vi "Populate.vi"(8 "error in":errorcluster, 9 "Values In":string[](array[string]), 10 "Keys In":string[](array[string]), 11 "Fast Tree in":refnum<class "Fast Tree.lvclass">) -> (0 "error out":errorcluster, 2 "Tree Out":T1(array[cluster]), 3 "Fast Tree out":refnum<class "Fast Tree.lvclass">)   [LabVIEW 2019, in "Fast Tree.lvclass"]
uses:
  Fast Tree.lvclass
  Fast Tree.lvclass/Fast Tree.ctl
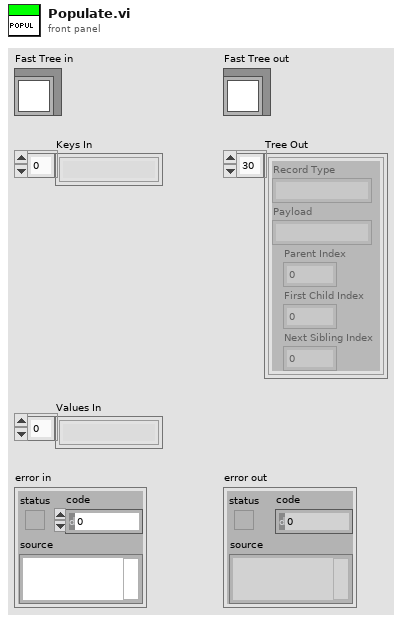
[diagram p1: front panel]
types:
  T1 = cluster{"Record Type":string, "Payload":string, "Parent Index":i32, "First Child Index":i32, "Next Sibling Index":i32}[]
  T2 = cluster{"Record Type":string, "Payload":string, "Parent Index":i32, "First Child Index":i32, "Next Sibling Index":i32}
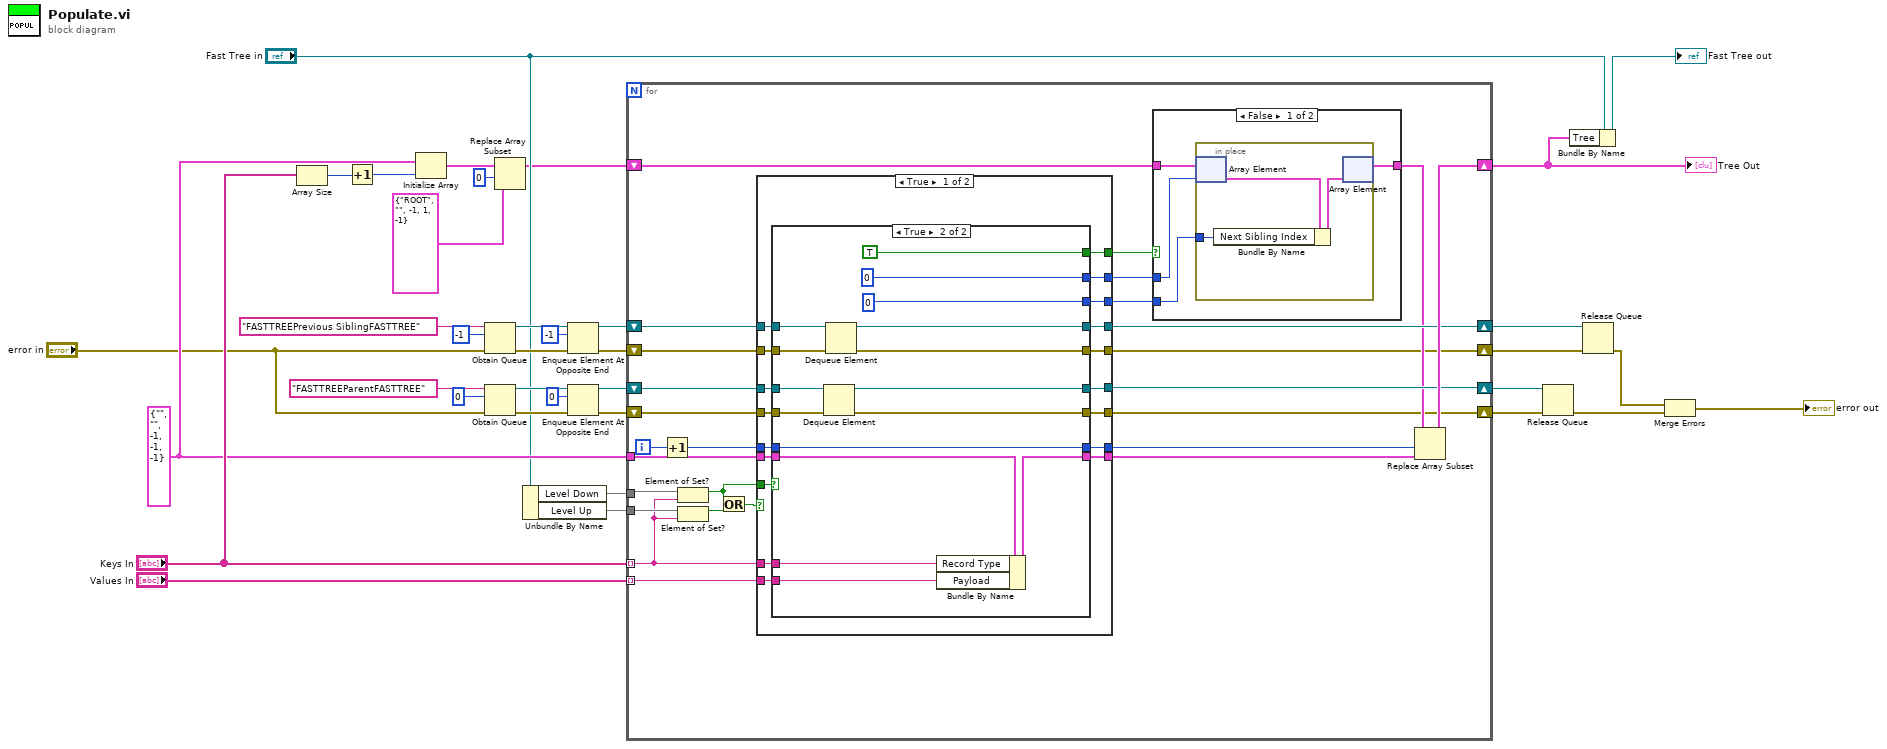
[diagram p0: block diagram]
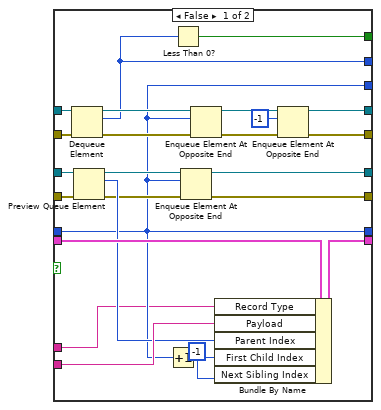
[diagram p3: hidden frame]
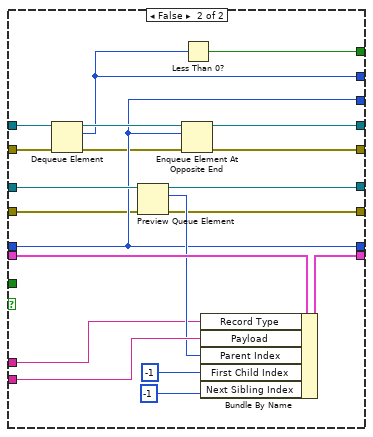
[diagram p4: hidden frame]
diagram:
  w17 = T2 {"Record Type"="", "Payload"="", "Parent Index"=-1, "First Child Index"=-1, "Next Sibling Index"=-1} ("Node")
  n1 = Array Size(array="Keys In") -> (size(s)=w18:i32)
  n2 = Increment(x=w18) -> (x+1=w11:i32)
  n3 = Initialize Array(w17, w11) -> (w10:T1)
  n4 = Obtain Queue(name (unnamed)="FASTTREEPrevious SiblingFASTTREE", element data type=-1, error in (no error)="error in") -> (queue out=w30:refnum<queue>, error out=w23:errorcluster)  [unwired: 2 in, 1 out]
  n5 = Obtain Queue(name (unnamed)="FASTTREEParentFASTTREE", element data type=0, error in (no error)="error in") -> (queue out=w32:refnum<queue>, error out=w22:errorcluster)  [unwired: 2 in, 1 out]
  n6 = Replace Array Subset(array=w10, new element=T2 {"Record Type"="ROOT", "Payload"="", "Parent Index"=-1, "First Child Index"=1, "Next Sibling Index"=-1} ("Node"), index=0) -> (w9:T1)
  n7 = Unbundle By Name("Fast Tree in") -> ("Level Down"=w15:set{string}, "Level Up"=w16:set{string})
  n8 = Enqueue Element At Opposite End(queue=w30, element=-1, error in (no error)=w23) -> (queue out=w26:refnum<queue>, error out=w24:errorcluster)  [unwired: 1 in, 1 out]
  n9 = Enqueue Element At Opposite End(queue=w32, element=0, error in (no error)=w22) -> (queue out=w31:refnum<queue>, error out=w21:errorcluster)  [unwired: 1 in, 1 out]
  n10 = for {
    shift-right: [w57] -> w12
    shift-left: w9 -> [w38]
    tunnel: "Keys In" -> [w40] mode=indexing
    tunnel: "Values In" -> [w61] mode=indexing
    tunnel: w17 -> [w62]
    shift-right: [w54] -> w35
    shift-left: w31 -> [w55]
    shift-right: [w52] -> w25
    shift-left: w26 -> [w53]
    shift-right: [w47] -> w5
    shift-left: w21 -> [w46]
    shift-right: [w45] -> w4
    shift-left: w24 -> [w44]
    tunnel: w16 -> [w43]
    tunnel: w15 -> [w42]
    i -> [w59]
    n11 = Increment(x=w59) -> (x+1=w58:i32)
    n12 = Element of Set?(10:w40, 11:w42) -> (3:w37:bool)
    n13 = Element of Set?(10:w40, 11:w43) -> (3:w41:bool)
    n14 = Or(x=w37, y=w41) -> (x .or. y?=w39:bool)
    n15 = case shown="True" w39 {
      tunnel: w62 -> [w86 w147]
      tunnel: w61 -> [w85 w146]
      tunnel: w58 -> [w79 w137]
      tunnel: [w87 w148] -> w60
      tunnel: [w73 w137] -> w56
      tunnel: w55 -> [w84 w145]
      tunnel: [w88 w140] -> w54
      tunnel: w53 -> [w83 w141]
      tunnel: [w82 w139] -> w52
      tunnel: [w81 w138] -> w48
      tunnel: [w80 w135] -> w50
      tunnel: [w72 w137] -> w49
      tunnel: [w77 w131] -> w47
      tunnel: w46 -> [w78 w130]
      tunnel: [w76 w132] -> w45
      tunnel: w44 -> [w75 w134]
      tunnel: w40 -> [w71 w129]
      tunnel: w37 -> [w74 _]
      frame True {
        n16 = case shown="True" w74 {
          tunnel: [w112 w118] -> w88
          tunnel: [w111 w116] -> w87
          tunnel: w86 -> [w110 w115]
          tunnel: w85 -> [w109 w113]
          tunnel: w84 -> [w107 w119]
          tunnel: w83 -> [w103 w128]
          tunnel: [w101 w125] -> w82
          tunnel: [w99 TRUE] -> w81
          tunnel: [w98 0] -> w80
          tunnel: w79 -> [w90 w122]
          tunnel: w78 -> [w96 w120]
          tunnel: [w94 w121] -> w77
          tunnel: [w93 w126] -> w76
          tunnel: w75 -> [w91 w127]
          tunnel: [w90 w122] -> w73
          tunnel: [w90 0] -> w72
          tunnel: w71 -> [w89 w114]
          frame False {
            n17 = Dequeue Element(queue=w103, error in (no error)=w91) -> (queue out=w104:refnum<queue>, element=w98:i32, error out=w92:errorcluster)  [unwired: 1 in, 1 out]
            n18 = Preview Queue Element(queue=w107, error in (no error)=w96) -> (queue out=w108:refnum<queue>, element=w97:i32, error out=w95:errorcluster)  [unwired: 1 in, 1 out]
            n19 = Increment(x=w90) -> (x+1=w106:i32)
            n20 = Less Than 0?(x=w98) -> (x < 0?=w99:bool)
            n21 = Enqueue Element At Opposite End(queue=w108, element=w90, error in (no error)=w95) -> (queue out=w112:refnum<queue>, error out=w94:errorcluster)  [unwired: 1 in, 1 out]
            n22 = Enqueue Element At Opposite End(queue=w104, element=w90, error in (no error)=w92) -> (queue out=w102:refnum<queue>, error out=w93:errorcluster)  [unwired: 1 in, 1 out]
            n23 = Bundle By Name(cluster=w110, "Record Type"=w89, "Payload"=w109, "Parent Index"=w97, "First Child Index"=w106, "Next Sibling Index"=-1) -> (w111:T2)
            n24 = Enqueue Element At Opposite End(queue=w102, element=-1) -> (queue out=w101:refnum<queue>)  [unwired: 2 in, 2 out]
          }
          frame True {
            n25 = Dequeue Element(queue=w119, error in (no error)=w120) -> (queue out=w118:refnum<queue>, error out=w121:errorcluster)  [unwired: 1 in, 2 out]
            n26 = Dequeue Element(queue=w128, error in (no error)=w127) -> (queue out=w125:refnum<queue>, error out=w126:errorcluster)  [unwired: 1 in, 2 out]
            n27 = Bundle By Name(cluster=w115, "Record Type"=w114, "Payload"=w113) -> (w116:T2)
          }
        }
      }
      frame False {
        n28 = Dequeue Element(queue=w141, error in (no error)=w134) -> (queue out=w142:refnum<queue>, element=w135:i32, error out=w133:errorcluster)  [unwired: 1 in, 1 out]
        n29 = Preview Queue Element(queue=w145, error in (no error)=w130) -> (queue out=w140:refnum<queue>, element=w144:i32, error out=w131:errorcluster)  [unwired: 1 in, 1 out]
        n30 = Enqueue Element At Opposite End(queue=w142, element=w137, error in (no error)=w133) -> (queue out=w139:refnum<queue>, error out=w132:errorcluster)  [unwired: 1 in, 1 out]
        n31 = Less Than 0?(x=w135) -> (x < 0?=w138:bool)
        n32 = Bundle By Name(cluster=w147, "Record Type"=w129, "Payload"=w146, "Parent Index"=w144, "First Child Index"=-1, "Next Sibling Index"=-1) -> (w148:T2)
      }
    }
    n33 = case shown="False" w48 {
      tunnel: [w65 w70] -> w51
      tunnel: w38 -> [w66 w70]
      tunnel: w49 -> [w64 _]
      tunnel: w50 -> [w63 _]
      frame False {
        n34 = in-place {
          in-place-border: w64 -> [w67]
          n35 = in-place-array #1(w66, w63) -> (w69:T2)
          n36 = Bundle By Name(cluster=w69, "Next Sibling Index"=w67) -> (w68:T2)
          n37 = in-place-array #1(w68) -> (w65:T1)  [unwired: 1 out]
        }
      }
      frame True {
      }
    }
    n38 = Replace Array Subset(array=w51, new element=w60, index=w56) -> (w57:T1)
  }
  "Tree Out" <- w12
  n39 = Release Queue(queue=w35, error in (no error)=w5) -> (error out=w1:errorcluster)  [unwired: 1 in, 2 out]
  n40 = Bundle By Name(cluster="Fast Tree in", "Tree"=w12) -> (→"Fast Tree out":refnum<class "Fast Tree.lvclass">)
  n41 = Release Queue(queue=w25, error in (no error)=w4) -> (error out=w3:errorcluster)  [unwired: 1 in, 2 out]
  n42 = Merge Errors(w3, w1) -> (→"error out":errorcluster)
